vi "myRIO_BRig_RT__testFPGA_sinwave.vi"() -> ()   [LabVIEW 2014]
uses:
  <vilib>/myRIO/Common/Instrument Driver Framework/myRIO v1.0/UART/vis/myRIO v1.0 Close UART.vi
  <vilib>/FPGAPlugInAG/myRIO-1900/niLvFpga_Open_myRIO-1900.vi
  <vilib>/rvi/interface/common/dynamic/niFpgaDynamicAddResources.vi
  <vilib>/Utility/error.llb/Error Cluster From Error Code.vi
  <vilib>/rvi/errors/niLvFpgaAdjustHostInterfaceError.vi
  <vilib>/FPGAPlugInAG/Dynamic/niLvFpga_Close_Dynamic.vi
  <vilib>/myRIO/Common/Instrument Driver Framework/Utilities/vis/FPGA Ref Manager.vi
  <vilib>/myRIO/Common/Instrument Driver Framework/myRIO v1.0/myRIO v1.0 Reset FPGA.vi
  <vilib>/myRIO/Common/Instrument Driver Framework/myRIO v1.0/IRQ/vis/myRIO v1.0 IRQ Info FGV.vi
  <vilib>/myRIO/Common/Instrument Driver Framework/myRIO v1.0/IRQ/vis/myRIO v1.0 Timer IRQ Info FGV.vi
  <vilib>/myRIO/Common/Instrument Driver Framework/myRIO v1.0/IRQ/vis/myRIO v1.0 ISR Agent.vi
  <vilib>/rvi/interface/nirviOpenFPGA/nirviOpenFPGA.xnode
  myRIO_BRig_FPGA_v3,51__build.lvbitx
  myRIO_BRig_FPGA_v3,51.vi
  <vilib>/rvi/interface/nirviReadWriteControl/nirviReadWriteControl.xnode
  <vilib>/rvi/interface/nirviCloseFPGA/nirviCloseFPGA.xnode
  NiFpgaLv.dll
  <vilib>/rvi/interface/Simulation/niFpgaSimulationCallBeginRW.vi
  <vilib>/myRIO/Instrument Drivers/Utilities/Utilities.lvlib
panel:
  out "Waveform Graph 2":i16[](graph)
  in  "k1_counts/ms":u16=159
  out "Waveform Graph":i16[](graph)
  out "Array":i16[][](array[numeric])
  out "duration [ms]":dbl
  in  "stop":bool
  in  "N":u16
  in  "audioTrigger_L":bool
  in  "audioTrigger_R":bool
  in  "audioFreq_L_kHz":u8=14 min=1 max=14 step=1
  in  "audioAmp_L":u16=1 min=1 max=32767 step=1
  in  "audioFreq_R_kHz":u8=14 min=1 max=14 step=1
  in  "audioAmp_R":u16=1 min=1 max=32767 step=1
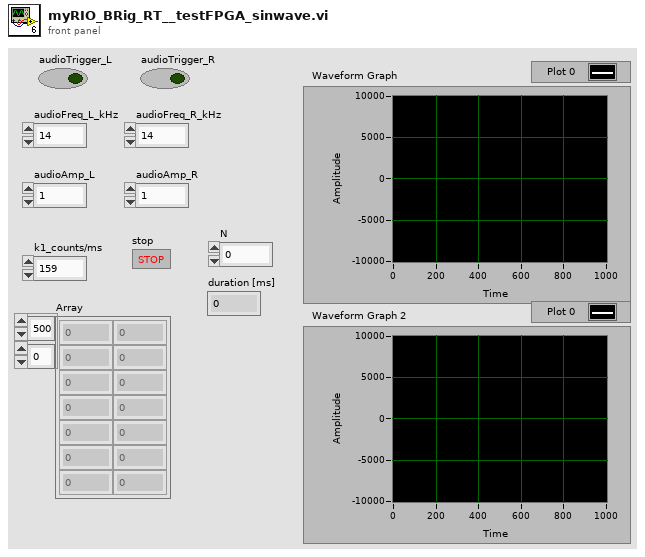
[diagram p1: front panel]
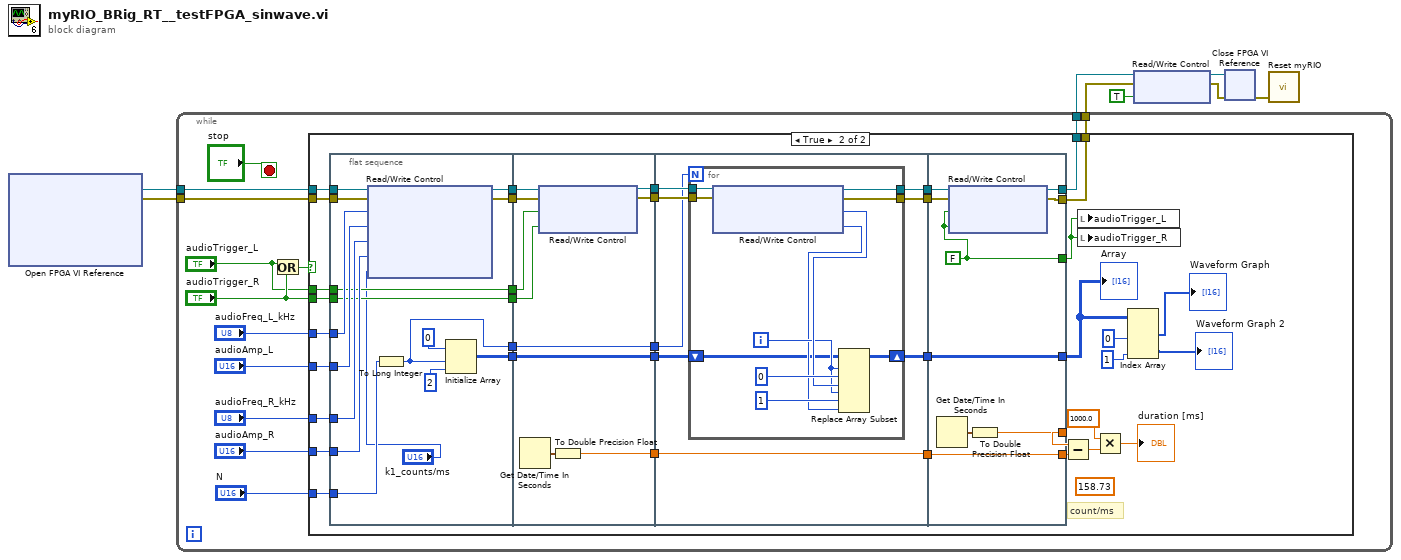
[diagram p0: block diagram]
diagram:
  n1 = xnode "Open FPGA VI Reference"() -> ("FPGA VI Reference Out"=w8:refnum<k20>, "error out"=w3:errorcluster)  [unwired: 2 in]
  n2 = while {
    tunnel: w8 -> [w20]
    tunnel: w3 -> [w18]
    tunnel: [w10] -> w2
    tunnel: [w9] -> w1
    stop <- "stop" stop-if-true
    n3 = Or(x="audioTrigger_L", y="audioTrigger_R") -> (x .or. y?=w13:bool)
    n4 = case shown="True" w13 {
      tunnel: "N" -> [_ w56]
      tunnel: w20 -> [w23 w55]
      tunnel: w18 -> [w22 w54]
      tunnel: "audioAmp_R" -> [_ w53]
      tunnel: "audioFreq_R_kHz" -> [_ w52]
      tunnel: "audioAmp_L" -> [_ w51]
      tunnel: "audioFreq_L_kHz" -> [_ w50]
      tunnel: "audioTrigger_R" -> [_ w48]
      tunnel: "audioTrigger_L" -> [_ w46]
      tunnel: [w23 w38] -> w10
      tunnel: [w22 w37] -> w9
      frame False {
      }
      frame True {
        (unwired) 158.73
        # "count/ms"
        n5 = flat-sequence {
          tunnel: w56 -> [w63]
          tunnel: [w75] -> w60
          tunnel: w55 -> [w74]
          tunnel: w54 -> [w73]
          tunnel: w53 -> [w72]
          tunnel: w52 -> [w71]
          tunnel: w51 -> [w70]
          tunnel: w50 -> [w69]
          tunnel: [w68] -> w49
          tunnel: w48 -> [w68]
          tunnel: [w67] -> w47
          tunnel: w46 -> [w67]
          tunnel: [w66] -> w45
          tunnel: [w65] -> w44
          tunnel: [w62] -> w30
          tunnel: w60 -> [w86]
          tunnel: [w86] -> w59
          tunnel: [w84] -> w58
          tunnel: w49 -> [w80]
          tunnel: w47 -> [w81]
          tunnel: w45 -> [w83]
          tunnel: w44 -> [w82]
          tunnel: [w79] -> w43
          tunnel: [w78] -> w42
          tunnel: [w77] -> w31
          tunnel: w30 -> [w77]
          tunnel: w59 -> [w88]
          tunnel: w58 -> [w94]
          tunnel: [w94] -> w57
          tunnel: w43 -> [w93]
          tunnel: w42 -> [w92]
          tunnel: [w91] -> w41
          tunnel: [w90] -> w40
          tunnel: [w87] -> w39
          tunnel: w31 -> [w89]
          tunnel: [w114] -> w36
          tunnel: w57 -> [w114]
          tunnel: [w112] -> w35
          tunnel: w41 -> [w111]
          tunnel: w40 -> [w110]
          tunnel: w39 -> [w109]
          tunnel: [w109] -> w28
          tunnel: [w108] -> w38
          tunnel: [w107] -> w37
          tunnel: [w106] -> w29
          frame #0 {
            n6 = xnode "Read/Write Control"("FPGA VI Reference In"=w74, "error in"=w73, "audioFreq_L_kHz"=w69, "audioAmp_L"=w70, "audioFreq_R_kHz"=w71, "audioAmp_R"=w72, "k1__counter_per_ms"="k1_counts/ms") -> ("FPGA VI Reference Out"=w66:refnum<k20>, "error out"=w65:errorcluster)
            n7 = To Long Integer(number=w63) -> (32bit integer=w62:i32)
            n8 = Initialize Array(i16 0 ("element"), w62, 2 ("dimension size")) -> (w75:i16[][])
          }
          frame #1 {
            n9 = Get Date/Time In Seconds() -> (seconds since 1Jan1904=w85:timestamp)
            n10 = xnode "Read/Write Control"("FPGA VI Reference In"=w83, "error in"=w82, "audioTrigger_L"=w81, "audioTrigger_R"=w80) -> ("FPGA VI Reference Out"=w79:refnum<k20>, "error out"=w78:errorcluster)
            n11 = To Double Precision Float(number=w85) -> (double precision float=w84:dbl)
          }
          frame #2 {
            n12 = for {
              N: w89 -> [_]
              tunnel: w93 -> [w105]
              tunnel: w92 -> [w104]
              tunnel: [w98] -> w91
              tunnel: [w97] -> w90
              shift-right: [w95] -> w87
              shift-left: w88 -> [w96]
              i -> [w101]
              n13 = xnode "Read/Write Control"("FPGA VI Reference In"=w105, "error in"=w104) -> ("FPGA VI Reference Out"=w98:refnum<k20>, "error out"=w97:errorcluster, "output_audioValue_L"=w102:i16, "output_audioValue_R"=w99:i16)
              n14 = Replace Array Subset(array=w96, new element #1=w102, index (row) #1=w101, index (col) #1=0 ("disabled index (col)"), new element #2=w99, index (row) #2=w101, index (col) #2=1 ("disabled index (col)")) -> (w95:i16[][])
            }
          }
          frame #3 {
            w106 = FALSE
            n15 = Get Date/Time In Seconds() -> (seconds since 1Jan1904=w113:timestamp)
            n16 = xnode "Read/Write Control"("FPGA VI Reference In"=w111, "error in"=w110, "audioTrigger_L"=w106, "audioTrigger_R"=w106) -> ("FPGA VI Reference Out"=w108:refnum<k20>, "error out"=w107:errorcluster)
            n17 = To Double Precision Float(number=w113) -> (double precision float=w112:dbl)
          }
        }
        n18 = Subtract(x=w35, y=w36) -> (x-y=w34:dbl)
        n19 = local write "audioTrigger_L"(w29) -> ()
        n20 = local write "audioTrigger_R"(w29) -> ()
        n21 = Multiply(x=1000.0, y=w34) -> (x*y=→"duration [ms]":dbl)
        n22 = Index Array(array=w28, index (col) #1=0 ("index (row)"), index (col) #2=1 ("index (col)")) -> (element #1=→"Waveform Graph":i16[], element #2=→"Waveform Graph 2":i16[])  [unwired: 2 in]
        "Array" <- w28
      }
    }
  }
  n23 = xnode "Read/Write Control"("FPGA VI Reference In"=w2, "error in"=w1, "FPGA_Stop"=TRUE) -> ("FPGA VI Reference Out"=w5:refnum<k20>, "error out"=w6:errorcluster)
  n24 = xnode "Close FPGA VI Reference"("FPGA VI Reference In"=w5, "error in"=w6) -> ("error out"=w4:errorcluster)
  n25 = call <vilib>:"Reset myRIO.vi"("error in (no error)"=w4) -> ()  [unwired: 10 in, 1 out]
